vi "Actual Replot.vi"(8 "error in (no error)":errorcluster, 11 "XY WFRM Plot in":refnum<class "XY WFRM Plot.lvclass">) -> (0 "error out":errorcluster, 3 "XY WFRM Plot out":refnum<class "XY WFRM Plot.lvclass">)   [LabVIEW 2016, in "XY WFRM Plot.lvclass"]
uses:
  XY WFRM Plot.lvclass
  C:/github/LabActor/Plots/Plot/Plot.lvclass
  Plot/Plot.lvclass/Plot.ctl
  XY WFRM Plot.lvclass/XY WFRM Plot.ctl
  Plot/Read Files.vi
  Plot/Plot.lvclass
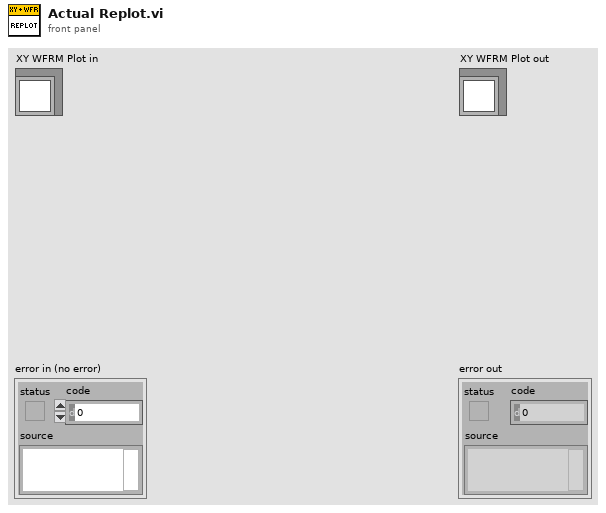
[diagram p1: front panel]
types:
  T1 = typedef "Plot types.ctl" = enum16{"Waveform Plot", "XY Plot", "Full XY"}
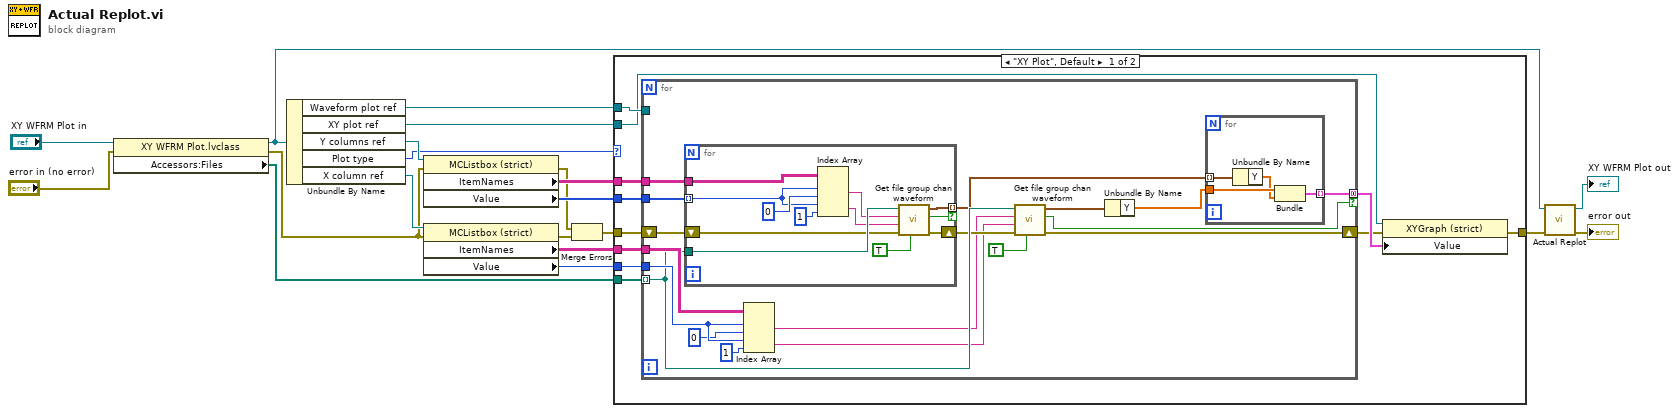
[diagram p0: block diagram]
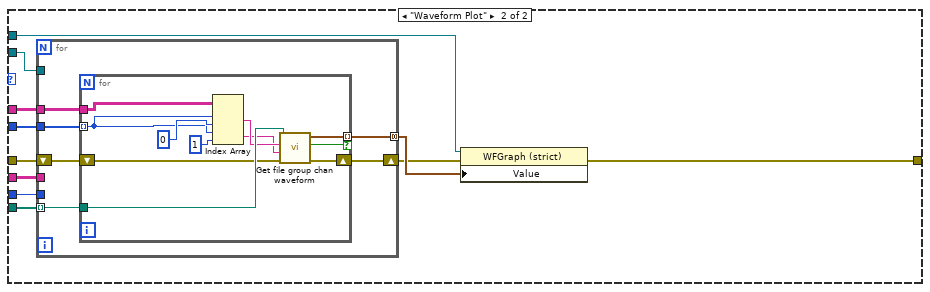
[diagram p2: hidden frame]
diagram:
  n1 = property class="XY WFRM Plot.lvclass"(reference="XY WFRM Plot in", error in="error in (no error)") -> (reference out=w2:refnum<class "XY WFRM Plot.lvclass">, error out=w9:errorcluster, "Accessors:Files"=w16:path[])
  n2 = Unbundle By Name(w2) -> ("Waveform plot ref"=w11:refnum<vi>, "XY plot ref"=w12:refnum<vi>, "Y columns ref"=w19:refnum<vi>, "Plot type"=w8:T1, "X column ref"=w15:refnum<vi>)
  n3 = property class="MCListbox (strict)"(reference=w19, error in=w9) -> (error out=w7:errorcluster, "ItemNames"=w18:string[][], "Value"=w17:i32[])  [unwired: 1 out]
  n4 = property class="MCListbox (strict)"(reference=w15, error in=w9) -> (error out=w6:errorcluster, "ItemNames"=w13:string[][], "Value"=w14:i32)  [unwired: 1 out]
  n5 = Merge Errors(w7, w6) -> (w5:errorcluster)
  n6 = case shown="\"XY Plot\", Default" w8 {
    tunnel: w18 -> [w31 w76]
    tunnel: w17 -> [w30 w75]
    tunnel: w16 -> [w29 w74]
    tunnel: w14 -> [w28 w73]
    tunnel: w13 -> [w27 w72]
    tunnel: w12 -> [w22 w71]
    tunnel: w11 -> [w26 w67]
    tunnel: [w23 w68] -> w4
    tunnel: w5 -> [w21 w66]
    frame "XY Plot", Default {
      n7 = for {
        tunnel: w31 -> [w49]
        tunnel: w30 -> [w48]
        tunnel: w29 -> [w44] mode=indexing
        shift-right: [w34] -> w24
        shift-left: w21 -> [w47]
        tunnel: w28 -> [w46]
        tunnel: w27 -> [w45]
        tunnel: w26 -> [_]
        tunnel: [w35] -> w25 mode=concatenating if=w33
        n8 = for {
          tunnel: w49 -> [w65]
          tunnel: w48 -> [w63] mode=indexing
          tunnel: w44 -> [w61]
          shift-right: [w56] -> w42
          shift-left: w47 -> [w58]
          tunnel: [w57] -> w43 mode=indexing if=w55
          n9 = Index Array(array=w65, index (row) #1=w63, index (col) #1=0 ("disabled index (col)"), index (row) #2=w63, index (col) #2=1 ("disabled index (col)")) -> (element #1=w60:string, element #2=w59:string)
          n10 = call "Get file group chan waveform.vi"("Clear missing ch err"=TRUE, "Error In"=w58, "Channel"=w59, "Group"=w60, "File"=w61) -> ("Error Out"=w56:errorcluster, "Valid WFRM"=w55:bool, "Waveform"=w57:waveform(sgl))  [unwired: 4 in]
        }
        n11 = Index Array(array=w45, index (row) #1=w46, index (col) #1=0 ("index (col)"), index (row) #2=w46, index (col) #2=1 ("index (col)")) -> (element #1=w39:string, element #2=w38:string)
        n12 = call "Get file group chan waveform.vi"("Clear missing ch err"=TRUE, "Error In"=w42, "Channel"=w38, "Group"=w39, "File"=w44) -> ("Error Out"=w34:errorcluster, "Valid WFRM"=w33:bool, "Waveform"=w37:waveform(sgl))  [unwired: 4 in]
        n13 = Unbundle By Name(w37) -> ("Y"=w36:sgl[])
        n14 = for {
          tunnel: w36 -> [w53]
          tunnel: w43 -> [w52] mode=indexing
          tunnel: [w50] -> w35 mode=indexing
          n15 = Unbundle By Name(w52) -> ("Y"=w51:sgl[])
          n16 = Bundle("Y"=w53, "Y"=w51) -> (w50:cluster{"Y":sgl[], "Y":sgl[]})  [unwired: 1 in]
        }
      }
      n17 = property class="XYGraph (strict)"(reference=w22, error in=w24, "Value"=w25) -> (error out=w23:errorcluster)  [unwired: 1 out]
    }
    frame "Waveform Plot" {
      n18 = for {
        tunnel: w76 -> [w82]
        tunnel: w75 -> [w81]
        tunnel: w74 -> [w79] mode=indexing
        shift-right: [w78] -> w69
        shift-left: w66 -> [w80]
        tunnel: w73 -> [_]
        tunnel: w72 -> [_]
        tunnel: w71 -> [_]
        tunnel: [w77] -> w70 mode=concatenating
        n19 = for {
          tunnel: w82 -> [w93]
          tunnel: w81 -> [w91] mode=indexing
          tunnel: w79 -> [w89]
          shift-right: [w85] -> w78
          shift-left: w80 -> [w86]
          tunnel: [w84] -> w77 mode=indexing if=w83
          n20 = Index Array(array=w93, index (row) #1=w91, index (col) #1=0 ("disabled index (col)"), index (row) #2=w91, index (col) #2=1 ("disabled index (col)")) -> (element #1=w88:string, element #2=w87:string)
          n21 = call "Get file group chan waveform.vi"("Error In"=w86, "Channel"=w87, "Group"=w88, "File"=w89) -> ("Error Out"=w85:errorcluster, "Valid WFRM"=w83:bool, "Waveform"=w84:waveform(sgl))  [unwired: 5 in]
        }
      }
      n22 = property class="WFGraph (strict)"(reference=w67, error in=w69, "Value"=w70) -> (error out=w68:errorcluster)  [unwired: 1 out]
    }
  }
  n23 = call-parent "Actual Replot.vi"("error in (no error)"=w4, "Plot in"=w2) -> ("error out"=→"error out":errorcluster, "Plot out"=→"XY WFRM Plot out":refnum<class "XY WFRM Plot.lvclass">)  [unwired: 8 in]
